vi "update read checkpoint.vi"(8 "error in (no error)":errorcluster, 10 "checkpoint_dir":string, 11 "spec_dir":string) -> (0 "error out":errorcluster)   [LabVIEW 2019, in "libCheckpointUpdate.lvlib"]
doc: "void update_read_checkpoint(const char* spec_dir, const char* checkpoint_dir);"
uses:
  libCheckpointUpdate.lvlib
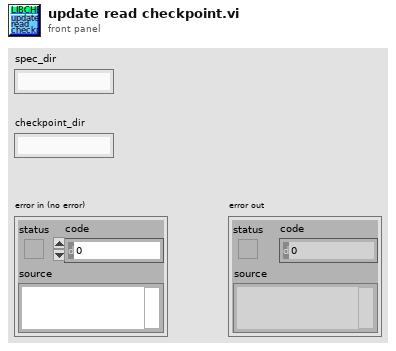
[diagram p1: front panel]
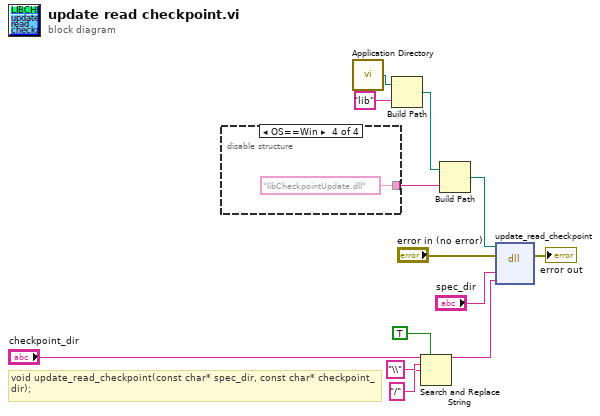
[diagram p0: block diagram]
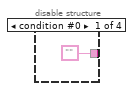
[diagram p2: hidden frame]
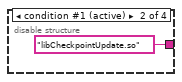
[diagram p3: hidden frame]
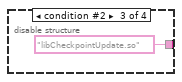
[diagram p4: hidden frame]
diagram:
  # "void update_read_checkpoint(const char* spec_dir, const char* checkpoint_dir);"
  n1 = disable-structure shown="OS==Win" {
    disable-tunnel: ["" "libCheckpointUpdate.so" ("name or relative path") "libCheckpointUpdate.so" ("name or relative path") "libCheckpointUpdate.dll" ("name or relative path")] -> w6
    frame condition #0 {
    }
    frame condition #1 (active) {
    }
    frame condition #2 {
    }
    frame condition #3 {
    }
  }
  n2 = call <vilib>:"Application Directory.vi"() -> ("Application Directory"=w10:path)
  n3 = Build Path(base path=w10, name or relative path="lib") -> (appended path=w8:path)
  n4 = Search and Replace String(replace all?=TRUE ("replace all? (F)"), input string="checkpoint_dir", search string="\\", replace string="/" ("replace string (\"\")")) -> (result string=w1:string)  [unwired: 4 in, 3 out]
  n5 = Build Path(base path=w8, name or relative path=w6) -> (appended path=w7:path)
  n6 = dll-call lib="home/paul/Schreibtisch/Biogas_plant_setup/LabView/lib/libCheckpointUpdate/libCheckpointUpdate.*" fn="update_read_checkpoint"(path in=w7, error in="error in (no error)", "spec_dir"="spec_dir", "checkpoint_dir"=w1) -> (error out=→"error out":errorcluster)  [unwired: 4 in, 1 out]
